vi "Windows Main.vi"() -> ()   [LabVIEW 2024]
panel:
  out "data out":waveform(dbl)(graph)
  in  "Folder to save file to":path=path "A:/Source Localization/Material Evaluation paper/Dataset/Microphone Characterization/Clean Source"
  in  "FileName":string
  in  "Stop Application":bool
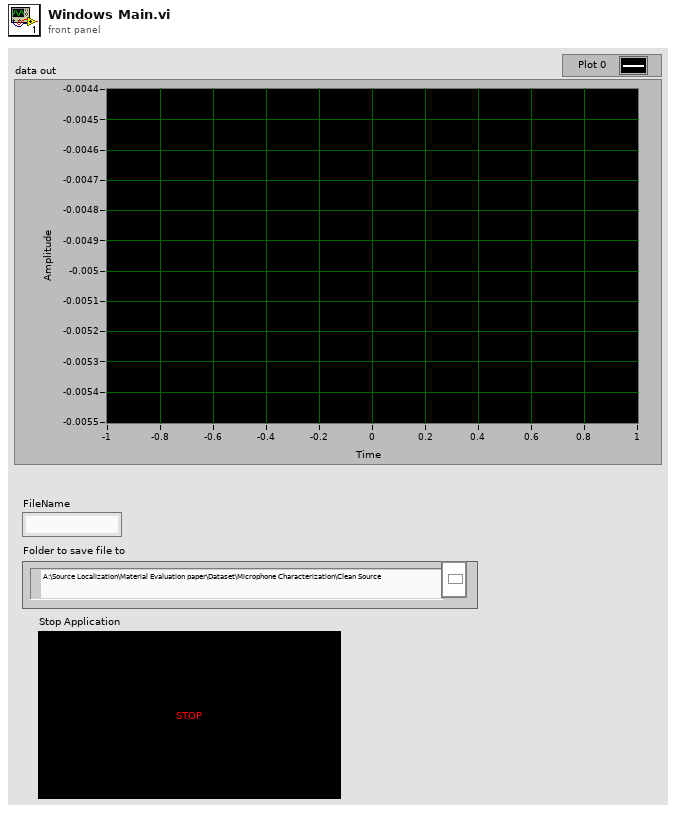
[diagram p1: front panel]
types:
  T1 = enum16{"open", "open or create", "create or replace", "create", "open (read-only)"}
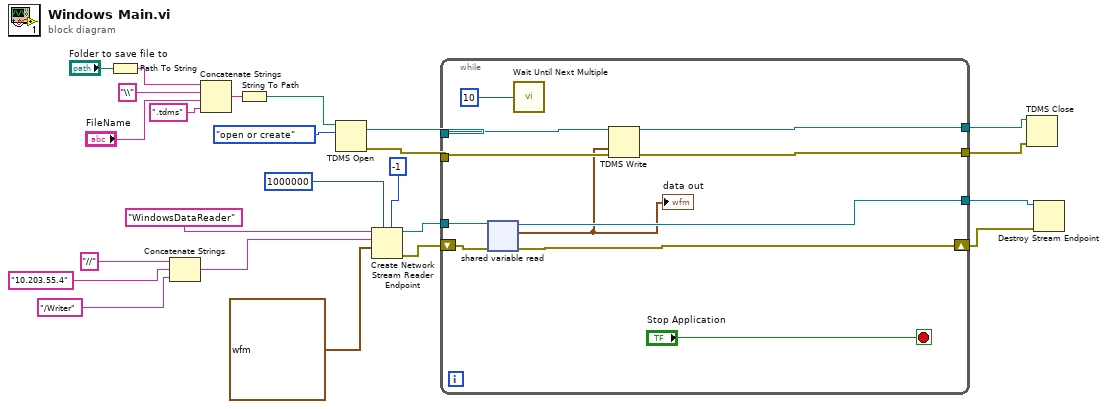
[diagram p0: block diagram]
diagram:
  n1 = Path To String(path="Folder to save file to") -> (string=w21:string)
  n2 = Concatenate Strings("//" ("string"), "10.203.55.4" ("string"), "/Writer" ("string")) -> (w9:string)
  n3 = Concatenate Strings(w21, "\\" ("string"), "FileName", ".tdms" ("string")) -> (w17:string)
  n4 = String To Path(string=w17) -> (path=w16:path)
  n5 = TDMS Open(10:T1."open or create" ("operation (0:open)"), 11:w16) -> (0:w14:errorcluster, 3:w15:refnum<k34>)  [unwired: 5 in]
  n6 = Create Network Stream Reader Endpoint(5:-1 ("timeout in ms (-1)"), 7:1000000 ("reader buffer size"), 9:waveform(dbl) {"t0"=timestamp(0 s since 1904-01-01), "dt"=1.0, "Y"=[]} ("Waveform"), 10:w9, 11:"WindowsDataReader" ("reader name")) -> (0:w24:errorcluster, 3:w23:refnum<k21>)  [unwired: 2 in]
  n7 = while {
    tunnel: w23 -> [w35]
    tunnel: [w31] -> w2
    shift-right: [w27] -> w3
    shift-left: w24 -> [w34]
    tunnel: w15 -> [w33]
    tunnel: w14 -> [w32]
    tunnel: [w30] -> w13
    tunnel: [w29] -> w4
    stop <- "Stop Application" stop-if-true
    n8 = shared-variable-read(w35, w34) -> (w31:refnum<k21>, w27:errorcluster, w25:waveform(dbl))  [unwired: 1 in, 1 out]
    "data out" <- w25
    n9 = call "Wait Until Next Multiple"("Count(Ticks)"=u32 10) -> ()  [unwired: 1 out]
    n10 = TDMS Write(0:w33, 9:w25, 11:w32) -> (4:w30:refnum<k34>, 15:w29:errorcluster)  [unwired: 3 in, 2 out]
  }
  n11 = TDMS Close(8:w4, 11:w13) -> ()  [unwired: 2 out]
  n12 = Destroy Stream Endpoint(8:w3, 11:w2) -> ()  [unwired: 1 out]
